vi "PS35_PosFEx.vi"(0 "Axis number":i32=1 min=1 max=3, 1 "Control unit ID":i32=1 min=1 max=10, 2 "dValue-In":dbl min=0.0 format="%.3f", 3 "error in (no error)":errorcluster, 5 "function":bool) -> (7 "dValue-Out":dbl format="%.3f", 9 "error out":errorcluster)   [LabVIEW 2020]
doc: "PS35_PosFEx.vi, created: 06.03.2009 alex; last change: 22.10.2019 alex;\n\n<B>FUNCTIONS:</B> \n\n<B>Read:</B> FALSE: read positioning velocity of an axis (values in selected unit).\n<B>Write:</B> TRUE: set positioning velocity of an axis (values in selected unit).\nIt is used for a trapezoidal and a S-curve profile.\nvelocity = unit/s\n----------------------------------------------------------------------------------------\n<B>INPUT:</B>\n[TF] <B>function:</B> function selector. (Read, Write)\n[I32] <B>Control unit ID:</B> control unit index. (Default=1, Range=1...10)\n[I32] <B>Axis number:</B> axis number. (Default=1, Range=1...3)\n[DBL] <B>dValue-In:</B> velocity value. (only for Write: Default=0.0)\n[CLU] <B>error in</B>\n----------------------------------------------------------------------------------------\n<B>OUTPUT:</B>\n[DBL] <B>dValue-Out:</B> velocity value. (for Write: dValue-Out=dValue-In)\n[CLU] <B>error out</B>\n----------------------------------------------------------------------------------------\n<B>SUB-VIs:</B>\nPS35_GetReadError.vi\n----------------------------------------------------------------------------------------\n<B>EXT-Calls:</B>\nps35.dll (V2.01)\n----------------------------------------------------------------------------------------"
uses:
  <vilib>/Utility/error.llb/DialogType.ctl
  ps35.dll
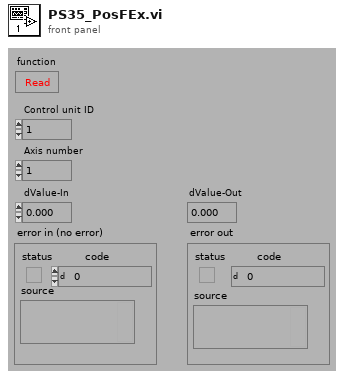
[diagram p1: front panel]
types:
  T1 = typedef "DialogType.ctl" = u16
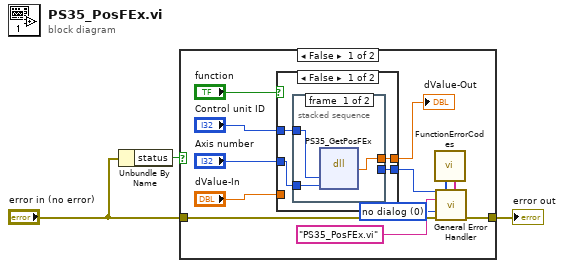
[diagram p0: block diagram]
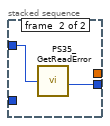
[diagram p2: hidden frame]
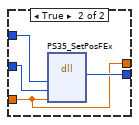
[diagram p3: hidden frame]
diagram:
  n1 = Unbundle By Name("error in (no error)") -> ("status"=w1:bool)
  n2 = case shown="False" w1 {
    tunnel: "error in (no error)" -> [w15 w29]
    tunnel: [w14 w29] -> w3
    frame False {
      w4 = T1 0 items=["no dialog", "OK message", "continue or stop message", "OK message + warnings", "continue/stop + warnings"] ("type of dialog (OK msg:1)")
      n3 = case shown="False" "function" {
        tunnel: "Control unit ID" -> [w18 w27]
        tunnel: [w19 w28] -> w11
        tunnel: "dValue-In" -> [_ w25]
        tunnel: [w17 w25] -> w9
        tunnel: "Axis number" -> [w16 w26]
        frame False {
          n4 = stacked-sequence {
            tunnel: [_ w24] -> w19
            tunnel: w18 -> [w22 w23]
            tunnel: [w21 _] -> w17
            tunnel: w16 -> [w20 _]
            frame #0 {
              n5 = dll-call lib="C:/GEECS/Developers Version/source/Device Drivers/OwiSoft_PS35/OWISoftOEM/ps35/labview/lv82/ps35.dll" fn="PS35_GetPosFEx" label="PS35_Get\nPosFEx"("Index"=w22, "AxisNr"=w20) -> ("Rückgabetyp"=w21:dbl)  [unwired: 5 in, 2 out]
            }
            frame #1 {
              n6 = call "PS35_GetReadError.vi"("Control unit ID"=w23) -> ("Read error"=w24:i32)
            }
          }
        }
        frame True {
          n7 = dll-call lib="C:/GEECS/Developers Version/source/Device Drivers/OwiSoft_PS35/OWISoftOEM/ps35/labview/lv82/ps35.dll" fn="PS35_SetPosFEx" label="PS35_Set\nPosFEx"("Index"=w27, "AxisNr"=w26, "dValue"=w25) -> ("Rückgabetyp"=w28:i32)  [unwired: 6 in, 2 out]
        }
      }
      "dValue-Out" <- w9
      n8 = call "FunctionErrorCodes.vi"() -> ("[user-defined codes]"=w5:i32[], "[user-defined descriptions]"=w6:string[])  [unwired: 8 in]
      n9 = call <vilib>:"General Error Handler.vi"("[error code] (0)"=w11, "[user-defined codes]"=w5, "[user-defined descriptions]"=w6, "[error source] (\" \")"="PS35_PosFEx.vi" ("[error source] (\" \")"), "type of dialog (OK msg:1)"=w4, "error in (no error)"=w15) -> ("error out"=w14:errorcluster)  [unwired: 5 in, 4 out]
    }
    frame True {
    }
  }
  "error out" <- w3
